vi "例4-19（1）.vi"() -> ()   [LabVIEW 2019]
panel:
  in  "停止":bool
  out "数值显示":dbl(knob) scale=0.0..10.0
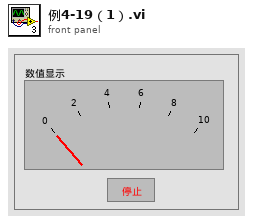
[diagram p1: front panel]
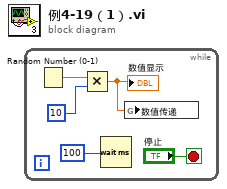
[diagram p0: block diagram]
diagram:
  n1 = while {
    stop <- "停止" stop-if-true
    n2 = Random Number (0-1)() -> (number: 0 to 1=w4:dbl)
    n3 = Multiply(x=w4, y=10) -> (x*y=w2:dbl)
    "数值显示" <- w2
    n4 = Wait (ms)(milliseconds to wait=100) -> ()  [unwired: 1 out]
    n5 = global write "例4-19（全局变量）.vi" "数值传递"(w2) -> ()
  }
